vi "Set Cell Value (Number).vi"(8 "error in":errorcluster, 9 "Number":string, 10 "Cell Address":string, 11 "WorksheetPart in":refnum<k24>) -> (0 "error out":errorcluster, 3 "WorksheetPart out":refnum<k24>)   [LabVIEW 2019, in "Open Xml.lvlib"]
uses:
  Open Xml.lvlib
  D:/git/Open-Xml-LabVIEW/Source/DocumentFormat.OpenXml.dll
  DocumentFormat.OpenXml.dll
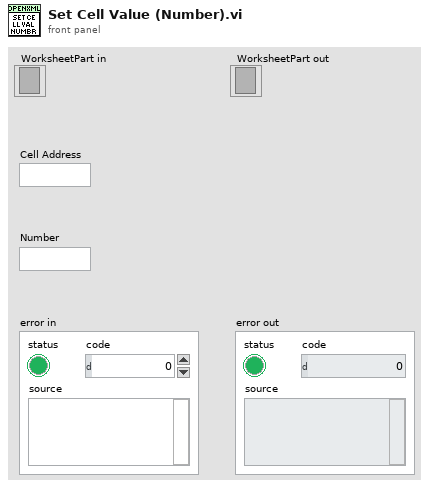
[diagram p1: front panel]
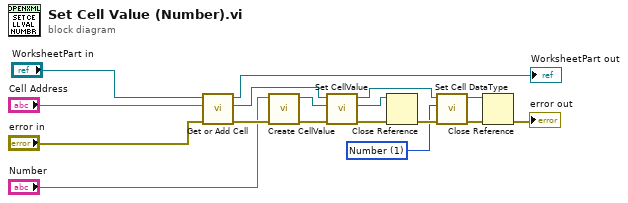
[diagram p0: block diagram]
diagram:
  w10 = 1 items=["Boolean", "Number", "Error", "SharedString", "String", "InlineString", "Date"] ("Datatype")
  n1 = call "Get or Add Cell.vi"("error in"="error in", "Cell Address"="Cell Address", "Worksheetpart in"="WorksheetPart in") -> ("error out"=w5:errorcluster, "Cell"=w12:refnum<k24>, "WorksheetPart out"=→"WorksheetPart out":refnum<k24>)  [unwired: 6 in]
  n2 = call "Create CellValue.vi"("error in"=w5, "Text"="Number") -> ("error out"=w6:errorcluster, "CellValue out"=w11:refnum<k24>)  [unwired: 8 in]
  n3 = call "Set CellValue.vi"("error in"=w6, "CellValue in"=w11, "Cell in"=w12) -> ("error out"=w9:errorcluster, "CellValue out"=w15:refnum<k24>, "Cell out"=w8:refnum<k24>)  [unwired: 6 in]
  n4 = Close Reference(reference=w15, error in (no error)=w9) -> (error out=w14:errorcluster)
  n5 = call "Set Cell DataType.vi"("error in"=w14, "Datatype"=w10, "Cell in"=w8) -> ("error out"=w7:errorcluster, "Cell out"=w17:refnum<k24>)  [unwired: 7 in]
  n6 = Close Reference(reference=w17, error in (no error)=w7) -> (error out=→"error out":errorcluster)
